vi "CmdExe.Launch Executable with Timeout, Abort, and Error Checks_V3a.vi"(4 "StdIn":string, 6 "Setup":T2={"Timeout (s)"=60.0, "Show Cmd Win"=FALSE, "Error Check"={"StdOut_Ck"=FALSE, "StdOutErrMsgs"=["Error", "Unable to find device "], "StdErr_Ck"=FALSE, "RtnCode_Ck"=FALSE, "RtnCodePASS"=0}, "Log_En"=FALSE, "LogFileName"="", "LogDir"=path ""}, 7 "CtrlRef":T1, 8 "error in (no error)":errorcluster, 9 "Ignore StdErr":bool, 10 "Args":string, 11 "Executable":path=path "C:/MTE/FW Load and Display Cal/Config/Bin/utahev_0_7/lighthouse_configtool.exe") -> (0 "error out":errorcluster, 1 "Duration(s)":dbl, 2 "return code":i32, 3 "Data Out":string)   [LabVIEW 2018]
uses:
  CmdExe.Setup Params.ctl
  CmdExe.Output Error Check Setup.ctl
  Errors/Error.Error Code List.ctl
  <vilib>/KATE/Time/Time Utils.lvlib
  <vilib>/KATE/Files/File Utils.lvlib
panel:
  out "Cmd":string
  out "Done":bool
  # "Launch Exe"
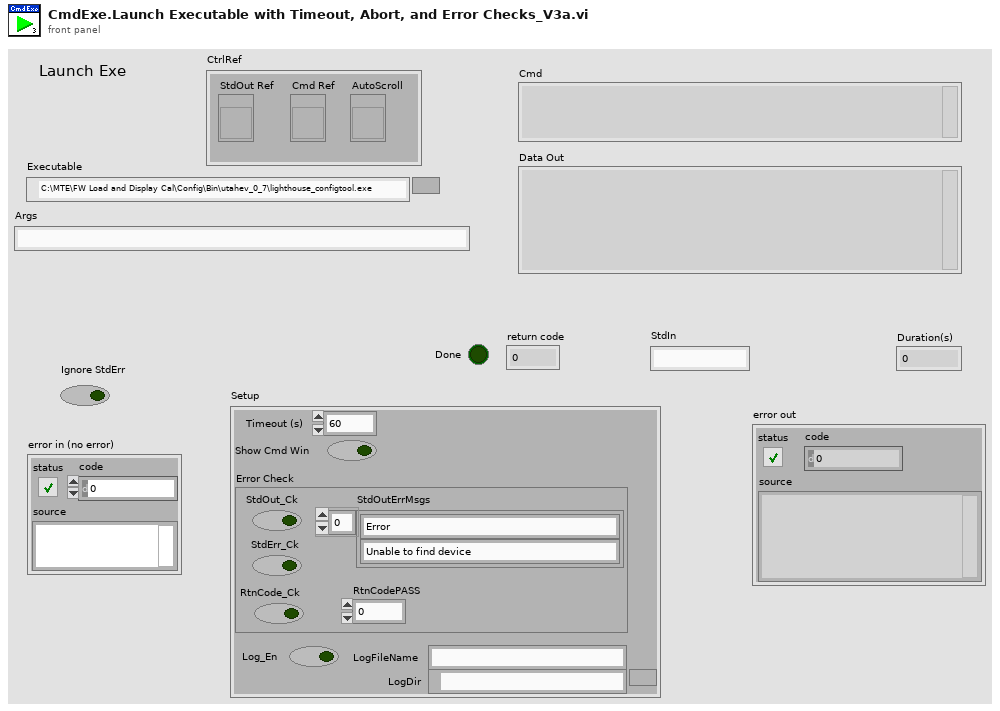
[diagram p1: front panel]
types:
  T1 = cluster{"StdOut Ref":refnum<vi>, "Cmd Ref":refnum<vi>, "AutoScroll":refnum<vi>}
  T2 = typedef "CmdExe.Setup Params.ctl" = cluster{"Timeout (s)":dbl, "Show Cmd Win":bool, "Error Check":T3, "Log_En":bool, "LogFileName":string, "LogDir":path}
  T3 = typedef "CmdExe.Output Error Check Setup.ctl" = cluster{"StdOut_Ck":bool, "StdOutErrMsgs":string[], "StdErr_Ck":bool, "RtnCode_Ck":bool, "RtnCodePASS":i32}
  T4 = enum16{"open", "replace", "create", "open or create", "replace or create", "replace or create with confirmation"}
  T5 = cluster{"Exe":string, "StdOut":string, "StdError":string, "LogFile":path, "Args":string, "TimedOut":bool, "RtnCode":i32, "LogEn":bool}
  T6 = typedef "Error.Error Code List.ctl" = i32
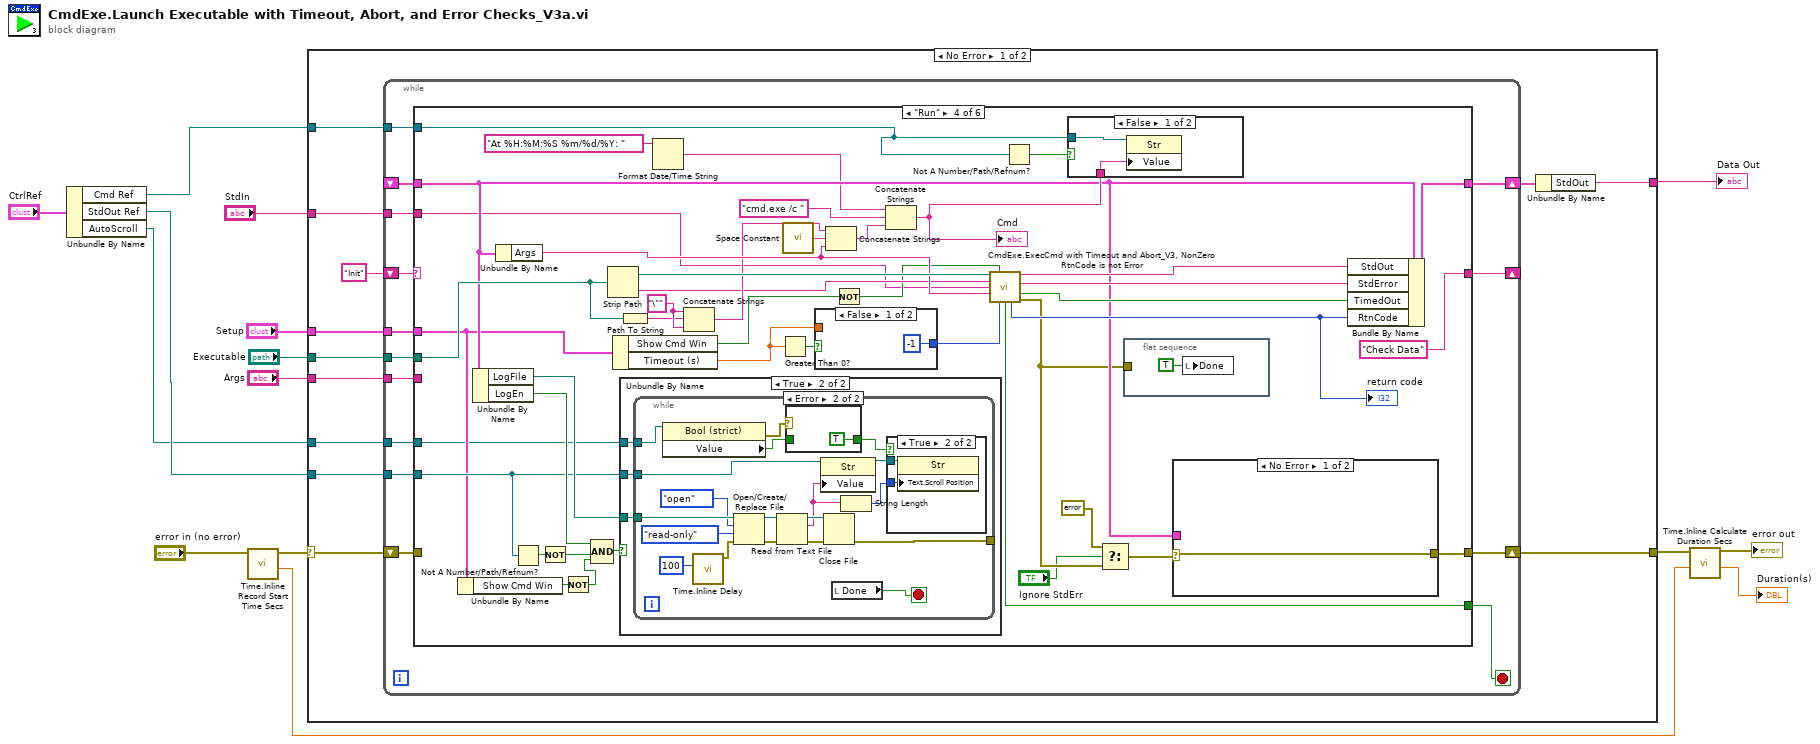
[diagram p0: block diagram]
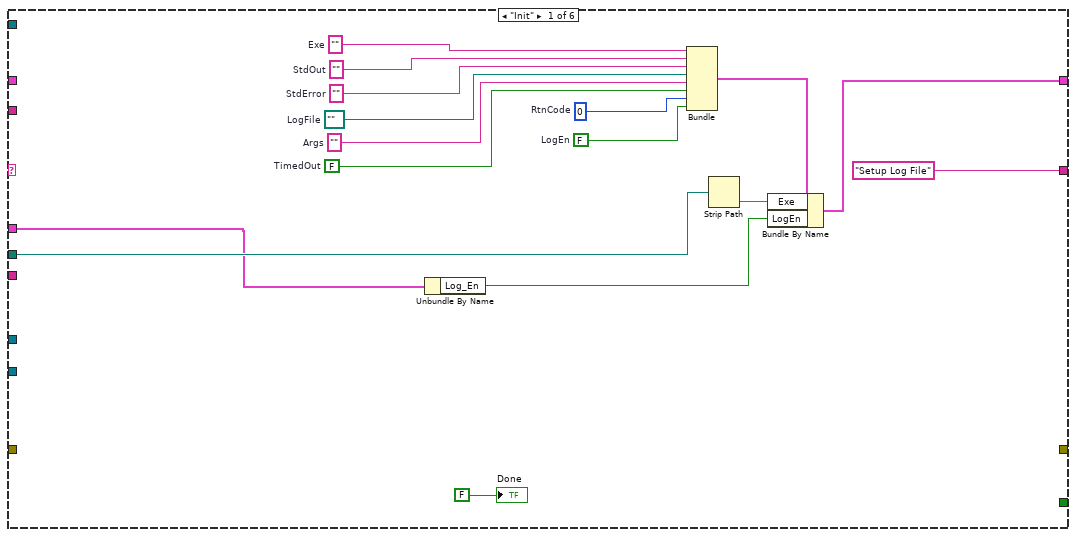
[diagram p2: hidden frame]
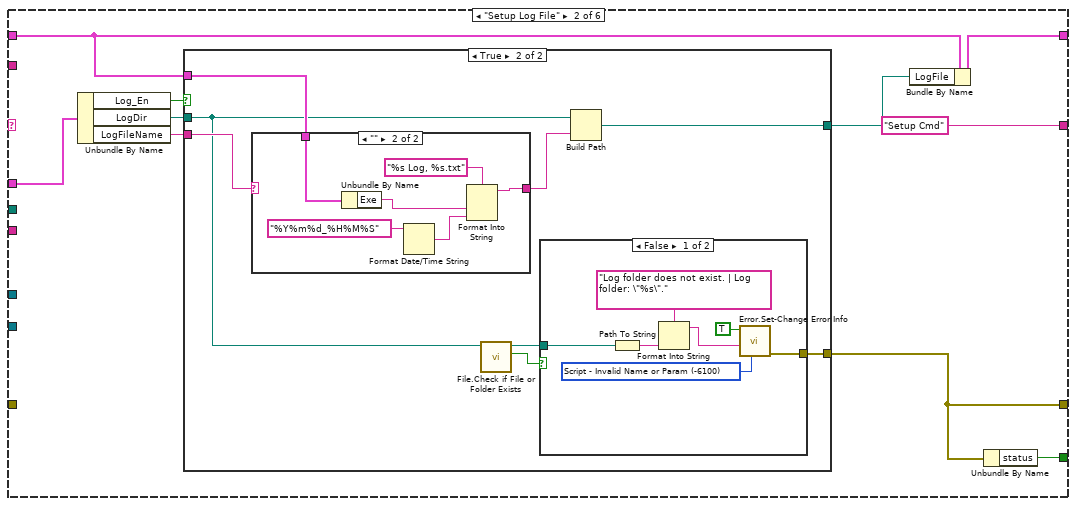
[diagram p3: hidden frame]
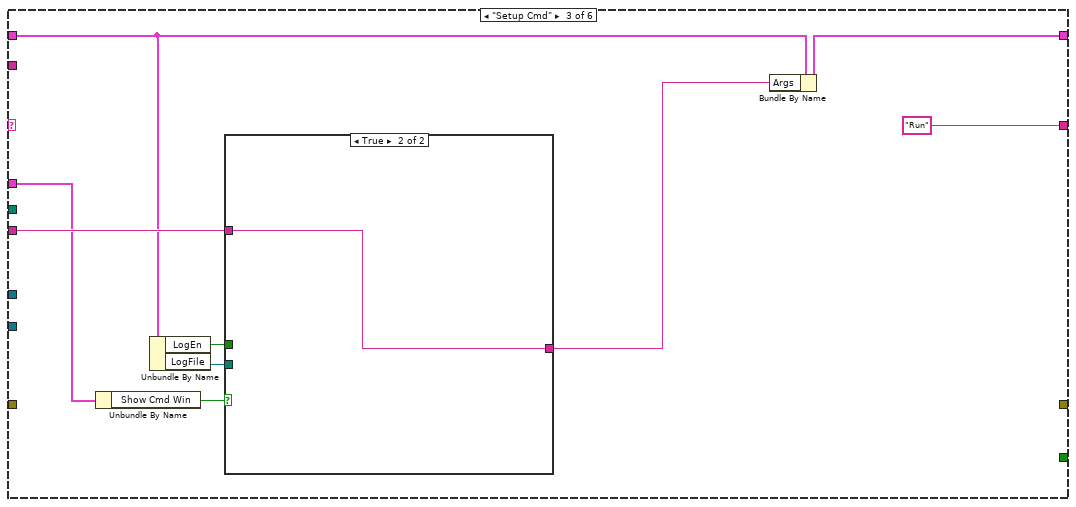
[diagram p7: hidden frame]
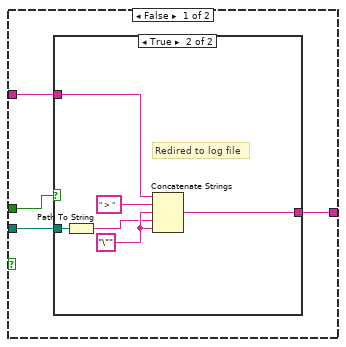
[diagram p8: hidden frame]
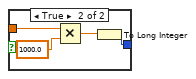
[diagram p10: hidden frame]
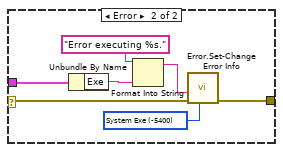
[diagram p11: hidden frame]
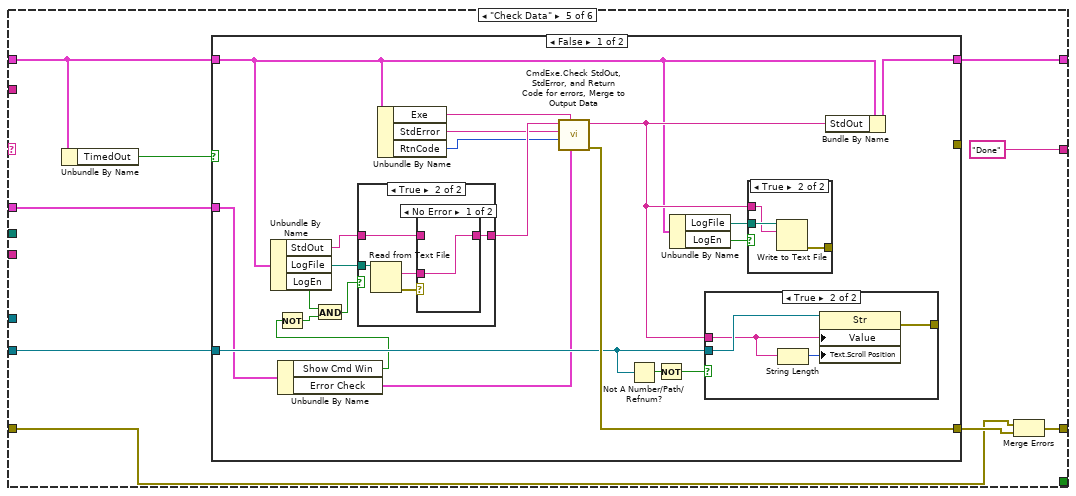
[diagram p16: hidden frame]
diagram:
  n1 = Unbundle By Name("CtrlRef") -> ("Cmd Ref"=w3:refnum<vi>, "StdOut Ref"=w2:refnum<vi>, "AutoScroll"=w1:refnum<vi>)
  n2 = call <vilib>:"Time.Inline Record Start Time Secs.vi"("Error In Upper"="error in (no error)") -> ("Start(s)"=w12:dbl, "Error Out Upper"=w15:errorcluster)  [unwired: 8 in, 1 out]
  n3 = case shown="No Error" w15 {
    selector: w15 -> [w26 w273]
    tunnel: [w25 w273] -> w14
    tunnel: [w23 _] -> w13
    tunnel: "Executable" -> [w22 _]
    tunnel: "Args" -> [w21 _]
    tunnel: "Setup" -> [w20 _]
    tunnel: w2 -> [w19 _]
    tunnel: "StdIn" -> [w18 _]
    tunnel: w3 -> [w17 _]
    tunnel: w1 -> [w16 _]
    frame No Error {
      n4 = while {
        shift-right: [w39] -> w24
        shift-left: _ -> [w38]
        shift-right: [w31] -> _
        shift-left: "Init" -> [w41]
        shift-right: [w37] -> w25
        shift-left: w26 -> [w40]
        tunnel: w22 -> [w35]
        tunnel: w21 -> [w34]
        tunnel: w20 -> [w33]
        tunnel: w19 -> [w32]
        tunnel: w18 -> [w30]
        tunnel: w17 -> [w29]
        tunnel: w16 -> [w28]
        stop <- w36 stop-if-true
        n5 = case shown="\"Run\"" w41 {
          tunnel: ["Setup Log File" "Setup Cmd" "Run" "Check Data" "Done" "Done"] -> w31
          tunnel: w40 -> [_ _ _ _ w197 w269]
          tunnel: [w46 w66 w97 w154 w205 w270] -> w39
          tunnel: [_ w59 _ w126 w199 w269] -> w37
          tunnel: w38 -> [_ w64 w92 w125 w203 w270]
          tunnel: [_ w58 _ w150 _ TRUE] -> w36
          tunnel: w35 -> [w49 _ _ w138 _ _]
          tunnel: w34 -> [_ _ w95 _ _ _]
          tunnel: w33 -> [w43 w63 w91 w120 w201 _]
          tunnel: w32 -> [_ _ _ w127 w204 _]
          tunnel: w30 -> [_ _ _ w117 _ _]
          tunnel: w29 -> [_ _ _ w114 _ _]
          tunnel: w28 -> [_ _ _ w113 _ _]
          frame "Init" {
            w44 = FALSE  # LogEn
            w45 = 0  # RtnCode
            w50 = FALSE  # TimedOut
            w51 = ""  # Args
            w52 = path ""  # LogFile
            w53 = ""  # StdError
            w54 = ""  # StdOut
            w56 = ""  # Exe
            n6 = Unbundle By Name(w43) -> ("Log_En"=w42:bool)
            n7 = Bundle("Exe"=w56, "StdOut"=w54, "StdError"=w53, "LogFile"=w52, "Args"=w51, "TimedOut"=w50, "RtnCode"=w45, "LogEn"=w44) -> (w47:T5)  [unwired: 1 in]
            n8 = Strip Path(path=w49) -> (name=w48:string)  [unwired: 1 out]
            n9 = Bundle By Name(cluster=w47, "Exe"=w48, "LogEn"=w42) -> (w46:T5)
            "Done" <- FALSE ("Done")
          }
          frame "Setup Log File" {
            n10 = Unbundle By Name(w63) -> ("Log_En"=w62:bool, "LogDir"=w61:path, "LogFileName"=w60:string)
            n11 = case shown="True" w62 {
              tunnel: [_ w75] -> w65
              tunnel: w64 -> [_ w73]
              tunnel: w61 -> [_ w69]
              tunnel: w60 -> [_ w72]
              tunnel: [_ w68] -> w59
              frame False {
              }
              frame True {
                n12 = case shown="\"\"" w72 {
                  selector: w72 -> [w83 _]
                  tunnel: [w83 w86] -> w74
                  tunnel: w73 -> [_ w85]
                  frame Default {
                  }
                  frame "" {
                    n13 = Unbundle By Name(w85) -> ("Exe"=w84:string)
                    n14 = Format Date/Time String(time format string (%c)="%Y%m%d_%H%M%S") -> (date/time string=w89:string)  [unwired: 2 in]
                    n15 = Format Into String(format string="%s Log, %s.txt", w84, w89) -> (resulting string=w86:string)  [unwired: 2 in, 1 out]
                  }
                }
                n16 = call <vilib>:"File.Check if File or Folder Exists.vi"("Path"=w69) -> ("Exists"=w70:bool, "Dup Path"=w71:path)  [unwired: 6 in, 3 out]
                n17 = case shown="False" w70 {
                  tunnel: [w76 _] -> w68
                  tunnel: w71 -> [w80 _]
                  frame False {
                    w78 = T6 -6100 items=["No Error"=0, "Abort"=-2, "Misc"=-5000, "Fixture Error"=-5100, "File IO - General"=-5200, "FIle IO - Config Error"=-5201, "Instrument - General"=-5300, "Instrument - Serial Com"=-5301, "Instrument - Camera"=-5302, "Instrument - PS"=-5303, "Instrument - Oscilloscope"=-5304, "Instrument - Function Gen"=-5305, "Instrument - Load"=-5306, "Instrument - Meter"=-5307, "Instrument - Power Control"=-5308, "Instrument - Motion"=-5309, "Instrument - RF"=-5310, "System Exe"=-5400, "Image Processing"=-5500, "Communication"=-5600, "Script - Syntax Error"=-6000, "Script - Invalid Name or Param"=-6100, "Script - Timeout"=-6200, "Invalid Data"=-6300] ("Std Code")
                    n18 = Path To String(path=w80) -> (string=w81:string)
                    n19 = Format Into String(format string="Log folder does not exist. | Log folder: \"%s\".", w81) -> (resulting string=w77:string)  [unwired: 2 in, 1 out]
                    n20 = call "Error.Set-Change Error Info.vi"("Std Code"=w78, "Description"=w77, "Set Error"=TRUE) -> ("error out"=w76:errorcluster)  [unwired: 8 in]
                  }
                  frame True {
                    # "Folders exist.\nNo error."
                  }
                }
                n21 = Build Path(base path=w69, name or relative path=w74) -> (appended path=w75:path)
              }
            }
            n22 = Bundle By Name(cluster=w64, "LogFile"=w65) -> (w66:T5)
            n23 = Unbundle By Name(w59) -> ("status"=w58:bool)
          }
          frame "Setup Cmd" {
            n24 = Unbundle By Name(w91) -> ("Show Cmd Win"=w90:bool)
            n25 = Unbundle By Name(w92) -> ("LogEn"=w93:bool, "LogFile"=w96:path)
            n26 = case shown="True" w90 {
              tunnel: w96 -> [w102 _]
              tunnel: w95 -> [w101 w110]
              tunnel: [w100 w110] -> w94
              tunnel: w93 -> [w99 _]
              frame False {
                n27 = case shown="True" w99 {
                  tunnel: w102 -> [_ w106]
                  tunnel: w101 -> [w103 w105]
                  tunnel: [w103 w104] -> w100
                  frame False {
                  }
                  frame True {
                    w109 = "\""
                    # "Redired to log file"
                    n28 = Path To String(path=w106) -> (string=w108:string)
                    n29 = Concatenate Strings(w105, " > ", w109, w108, w109) -> (w104:string)
                  }
                }
              }
              frame True {
              }
            }
            n30 = Bundle By Name(cluster=w92, "Args"=w94) -> (w97:T5)
          }
          frame "Run" {
            w139 = "\""
            n31 = Unbundle By Name(w120) -> ("Show Cmd Win"=w119:bool)
            n32 = Unbundle By Name(w125) -> ("LogFile"=w147:path, "LogEn"=w131:bool)
            n33 = Unbundle By Name(w125) -> ("Args"=w140:string)
            n34 = Not A Number/Path/Refnum?(number/path/refnum=w127) -> (NaN/Path/Refnum?=w134:bool)
            n35 = Not(x=w134) -> (.not. x?=w133:bool)
            n36 = Not(x=w119) -> (.not. x?=w118:bool)
            n37 = Compound Arithmetic op=AND(w131, w133, w118) -> (w132:bool)
            n38 = Strip Path(path=w138) -> (stripped path=w146:path, name=w135:string)
            n39 = Unbundle By Name(w120) -> ("Show Cmd Win"=w130:bool, "Timeout (s)"=w112:dbl)
            n40 = Path To String(path=w138) -> (string=w137:string)
            n41 = case shown="True" w132 {
              tunnel: w147 -> [_ w172]
              tunnel: w127 -> [_ w173]
              tunnel: w113 -> [_ w171]
              frame False {
              }
              frame True {
                n42 = while {
                  tunnel: w173 -> [w184]
                  tunnel: w172 -> [w188]
                  tunnel: [w187] -> _
                  tunnel: w171 -> [w178]
                  stop <- w183 stop-if-true
                  n43 = property class="Bool (strict)"(reference=w178) -> (error out=w176:errorcluster, "Value"=w175:bool)  [unwired: 1 in, 1 out]
                  n44 = call <vilib>:"Time.Inline Delay.vi"("Wait(ms)"=u32 100) -> ("error out top"=w181:errorcluster)  [unwired: 9 in, 1 out]
                  n45 = Open/Create/Replace File(file path (use dialog)=w188, error in=w181, operation (0:open)=T4."open", access (0:read/write)=enum16{"read/write", "read-only", "write-only"}."read-only") -> (refnum out=w189:refnum<file>, error out=w192:errorcluster)  [unwired: 2 in, 1 out]
                  n46 = Read from Text File(file (use dialog)=w189, error in=w192) -> (refnum out=w190:refnum<file>, text=w179:string, error out=w191:errorcluster)  [unwired: 2 in, 1 out]
                  n47 = case shown="Error" w176 {
                    tunnel: w175 -> [w193 _]
                    tunnel: [w193 TRUE ("Value")] -> w174
                    frame No Error {
                    }
                    frame Error {
                    }
                  }
                  n48 = property class="Str"(reference=w184, "Value"=w179) -> (reference out=w180:refnum<vi>)  [unwired: 1 in, 1 out]
                  n49 = Close File(refnum=w190, error in=w191) -> (error out=w187:errorcluster)  [unwired: 1 out]
                  n50 = local read "Done"() -> (w183:bool)
                  n51 = String Length(string=w179) -> (length=w177:i32)
                  n52 = case shown="True" w174 {
                    tunnel: w180 -> [_ w196]
                    tunnel: w177 -> [_ w195]
                    frame False {
                    }
                    frame True {
                      n53 = property class="Str"(reference=w196, "Text.Scroll Position"=w195) -> ()  [unwired: 1 in, 2 out]
                    }
                  }
                }
              }
            }
            n54 = Format Date/Time String(time format string (%c)="At %H:%M:%S %m/%d/%Y: ") -> (date/time string=w115:string)  [unwired: 2 in]
            n55 = Concatenate Strings(w139, w137, w139) -> (w136:string)
            n56 = Greater Than 0?(x=w112) -> (x > 0?=w111:bool)
            n57 = call <vilib>:"Space Constant.vi"() -> ("String"=w143:string)
            n58 = case shown="False" w111 {
              tunnel: [-1 w157] -> w149
              tunnel: w112 -> [_ w156]
              frame False {
              }
              frame True {
                n59 = Multiply(x=w156, y=1000.0) -> (x*y=w159:dbl)
                n60 = To Long Integer(number=w159) -> (32bit integer=w157:i32)
              }
            }
            n61 = Concatenate Strings(w136, w143, w140) -> (w144:string)
            n62 = Not(x=w130) -> (.not. x?=w129:bool)
            n63 = Concatenate Strings(w115, "cmd.exe /c ", w144) -> (w142:string)
            "Cmd" <- w142
            n64 = call "CmdExe.ExecCmd with Timeout and Abort_V3, NonZero RtnCode is not Error.vi"("Working Dir"=w146, "Run minimized? (T)"=w129, "Executable"=w135, "StdIn"=w117, "Arguements"=w140, "Timeout ms(-1)"=w149) -> ("STD OUT"=w128:string, "STD ERR"=w153:string, "Timed Out"=w152:bool, "Aborted"=w150:bool, "return code"=w141:i32, "error out"=w124:errorcluster)  [unwired: 4 in]
            "return code" <- w141
            n65 = Not A Number/Path/Refnum?(number/path/refnum=w114) -> (NaN/Path/Refnum?=w148:bool)
            n66 = case shown="False" w148 {
              tunnel: w114 -> [w170 _]
              tunnel: w142 -> [w169 _]
              frame False {
                n67 = property class="Str"(reference=w170, "Value"=w169) -> ()  [unwired: 1 in, 2 out]
              }
              frame True {
              }
            }
            n68 = Select(t=errorcluster {"status"=FALSE, "code"=0, "source"=""}, s="Ignore StdErr", f=w124) -> (s? t:f=w123:errorcluster)
            n69 = flat-sequence {
              tunnel: w124 -> [_]
              frame #0 {
                n70 = local write "Done"(TRUE ("Done")) -> ()
              }
            }
            n71 = case shown="No Error" w123 {
              selector: w123 -> [w160 w163]
              tunnel: [w160 w162] -> w126
              tunnel: w125 -> [_ w161]
              frame No Error {
              }
              frame Error {
                w165 = T6 -5400 items=["No Error"=0, "Abort"=-2, "Misc"=-5000, "Fixture Error"=-5100, "File IO - General"=-5200, "FIle IO - Config Error"=-5201, "Instrument - General"=-5300, "Instrument - Serial Com"=-5301, "Instrument - Camera"=-5302, "Instrument - PS"=-5303, "Instrument - Oscilloscope"=-5304, "Instrument - Function Gen"=-5305, "Instrument - Load"=-5306, "Instrument - Meter"=-5307, "Instrument - Power Control"=-5308, "Instrument - Motion"=-5309, "Instrument - RF"=-5310, "System Exe"=-5400, "Image Processing"=-5500, "Communication"=-5600, "Script - Syntax Error"=-6000, "Script - Invalid Name or Param"=-6100, "Script - Timeout"=-6200, "Invalid Data"=-6300] ("Std Code")
                n72 = Unbundle By Name(w161) -> ("Exe"=w166:string)
                n73 = Format Into String(format string="Error executing %s.", w166) -> (resulting string=w164:string)  [unwired: 2 in, 1 out]
                n74 = call "Error.Set-Change Error Info.vi"("Std Code"=w165, "error in"=w163, "Description"=w164) -> ("error out"=w162:errorcluster)  [unwired: 8 in]
              }
            }
            n75 = Bundle By Name(cluster=w125, "StdOut"=w128, "StdError"=w153, "TimedOut"=w152, "RtnCode"=w141) -> (w154:T5)
          }
          frame "Check Data" {
            n76 = Unbundle By Name(w203) -> ("TimedOut"=w202:bool)
            n77 = case shown="False" w202 {
              tunnel: [w226 w248] -> w205
              tunnel: w203 -> [w210 w242]
              tunnel: [w221 w253] -> w198
              tunnel: w204 -> [w218 _]
              tunnel: w201 -> [w215 w258]
              tunnel: [_ w243] -> _
              frame False {
                n78 = Unbundle By Name(w210) -> ("StdOut"=w216:string, "LogFile"=w225:path, "LogEn"=w209:bool)
                n79 = Unbundle By Name(w215) -> ("Show Cmd Win"=w207:bool, "Error Check"=w214:T3)
                n80 = Not(x=w207) -> (.not. x?=w208:bool)
                n81 = And(x=w209, y=w208) -> (x .and. y?=w206:bool)
                n82 = case shown="True" w206 {
                  tunnel: w225 -> [_ w239]
                  tunnel: [w234 w237] -> w224
                  tunnel: w216 -> [w234 w235]
                  frame False {
                    (unwired) TRUE
                  }
                  frame True {
                    n83 = Read from Text File(file (use dialog)=w239) -> (text=w236:string, error out=w238:errorcluster)  [unwired: 3 in, 2 out]
                    n84 = case shown="No Error" w238 {
                      tunnel: [w240 w241] -> w237
                      tunnel: w236 -> [w240 _]
                      tunnel: w235 -> [_ w241]
                      frame No Error {
                      }
                      frame Error {
                      }
                    }
                  }
                }
                n85 = Unbundle By Name(w210) -> ("Exe"=w217:string, "StdError"=w223:string, "RtnCode"=w222:i32)
                n86 = call "CmdExe.Check StdOut, StdError, and Return Code for errors, Merge to Output Data.vi"("Error Check"=w214, "App Name"=w217, "Return Code"=w222, "StdError"=w223, "StdOut"=w224) -> ("error out"=w221:errorcluster, "Output Data"=w211:string)  [unwired: 5 in]
                n87 = Not A Number/Path/Refnum?(number/path/refnum=w218) -> (NaN/Path/Refnum?=w220:bool)
                n88 = Not(x=w220) -> (.not. x?=w219:bool)
                n89 = Unbundle By Name(w210) -> ("LogFile"=w213:path, "LogEn"=w212:bool)
                n90 = case shown="True" w219 {
                  tunnel: w218 -> [_ w232]
                  tunnel: w211 -> [_ w231]
                  tunnel: [_ w230] -> _
                  frame False {
                  }
                  frame True {
                    n91 = String Length(string=w231) -> (length=w233:i32)
                    n92 = property class="Str"(reference=w232, "Value"=w231, "Text.Scroll Position"=w233) -> (error out=w230:errorcluster)  [unwired: 1 in, 1 out]
                  }
                }
                n93 = case shown="True" w212 {
                  tunnel: w213 -> [_ w229]
                  tunnel: [_ w228] -> _
                  tunnel: w211 -> [_ w227]
                  frame False {
                    (unwired) TRUE
                  }
                  frame True {
                    n94 = Write to Text File(file (use dialog)=w229, text=w227) -> (error out=w228:errorcluster)  [unwired: 2 in, 2 out]
                  }
                }
                n95 = Bundle By Name(cluster=w210, "StdOut"=w211) -> (w226:T5)
              }
              frame True {
                w256 = T6 -5400 items=["No Error"=0, "Abort"=-2, "Misc"=-5000, "Fixture Error"=-5100, "File IO - General"=-5200, "FIle IO - Config Error"=-5201, "Instrument - General"=-5300, "Instrument - Serial Com"=-5301, "Instrument - Camera"=-5302, "Instrument - PS"=-5303, "Instrument - Oscilloscope"=-5304, "Instrument - Function Gen"=-5305, "Instrument - Load"=-5306, "Instrument - Meter"=-5307, "Instrument - Power Control"=-5308, "Instrument - Motion"=-5309, "Instrument - RF"=-5310, "System Exe"=-5400, "Image Processing"=-5500, "Communication"=-5600, "Script - Syntax Error"=-6000, "Script - Invalid Name or Param"=-6100, "Script - Timeout"=-6200, "Invalid Data"=-6300] ("Std Code")
                n96 = Unbundle By Name(w258) -> ("Timeout (s)"=w257:dbl)
                n97 = Unbundle By Name(w242) -> ("StdOut"=w245:string, "LogFile"=w247:path, "LogEn"=w246:bool)
                n98 = Unbundle By Name(w242) -> ("Exe"=w259:string)
                n99 = Unbundle By Name(w242) -> ("Exe"=w250:string, "StdError"=w252:string, "RtnCode"=w251:i32)
                n100 = case shown="True" w246 {
                  tunnel: w247 -> [_ w266]
                  tunnel: [w261 w264] -> w244
                  tunnel: w245 -> [w261 w262]
                  frame False {
                    (unwired) TRUE
                  }
                  frame True {
                    n101 = Read from Text File(file (use dialog)=w266) -> (text=w263:string, error out=w265:errorcluster)  [unwired: 3 in, 2 out]
                    n102 = case shown="No Error" w265 {
                      tunnel: [w267 w268] -> w264
                      tunnel: w263 -> [w267 _]
                      tunnel: w262 -> [_ w268]
                      frame No Error {
                      }
                      frame Error {
                      }
                    }
                  }
                }
                n103 = Format Into String(format string="%s was terminated due to timeout (%.1f secs).  ", w259, w257) -> (resulting string=w254:string)  [unwired: 2 in, 1 out]
                n104 = call "CmdExe.Check StdOut, StdError, and Return Code for errors, Merge to Output Data.vi"("App Name"=w250, "Return Code"=w251, "StdError"=w252, "StdOut"=w244) -> ("error out"=w243:errorcluster, "Output Data"=w249:string)  [unwired: 6 in]
                n105 = call "Error.Set-Change Error Info.vi"("Std Code"=w256, "Description"=w254, "Set Error"=TRUE) -> ("error out"=w253:errorcluster)  [unwired: 8 in]
                n106 = Bundle By Name(cluster=w242, "StdOut"=w249) -> (w248:T5)
              }
            }
            n107 = Merge Errors(w197, w198) -> (w199:errorcluster)
          }
          frame "Done", Default {
          }
        }
      }
      n108 = Unbundle By Name(w24) -> ("StdOut"=w23:string)
    }
    frame Error {
    }
  }
  "Data Out" <- w13
  n109 = call <vilib>:"Time.Inline Calculate Duration Secs.vi"("Start(Sec)"=w12, "Error In Top"=w14) -> ("Duration(s)"=→"Duration(s)":dbl, "Error Out Top"=→"error out":errorcluster)  [unwired: 7 in, 1 out]
